vi "Dynamixel Read Pos.vi"(11 "Com port":refnum<visa-resource-name> caption="instrument handle") -> ()   [LabVIEW 2022 SP3]
uses:
  Library/dxl_x64_c.lvlib
  Sub Vis/Dynamixel Commands.ctl
panel:
  in  "Function":T1
  out "value : PRO (knob)\npresent position":i32(knob) scale=150000.0..-150000.0
  in  "protocol_version":i32=2
  out "port_num":i32
  in  "dynamixel_id":u8=1
  in  "baud_rate":i32=57600
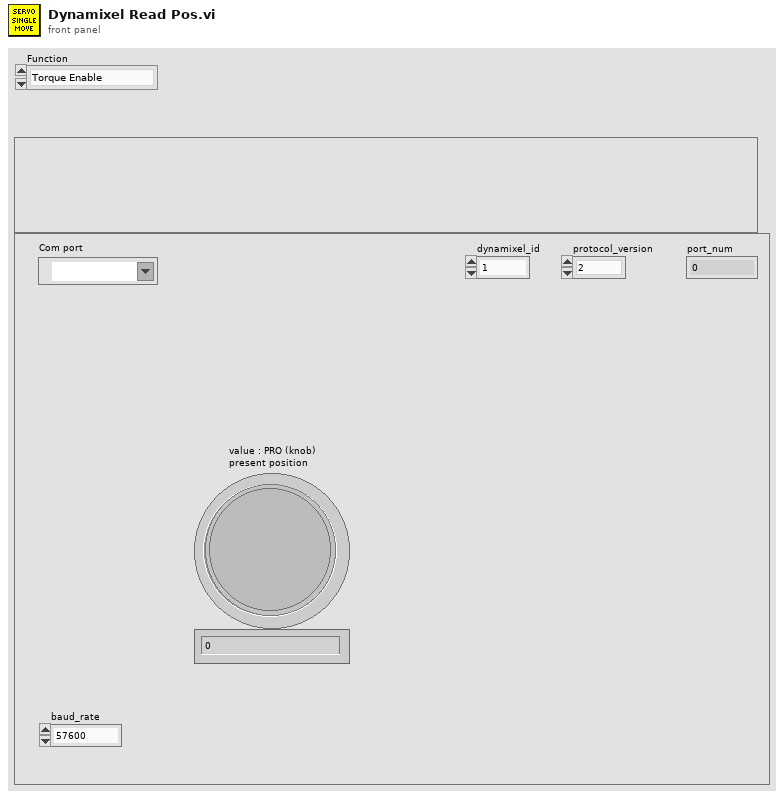
[diagram p1: front panel]
types:
  T1 = typedef "Dynamixel Commands.ctl" = enum16{"Torque Enable", "Present Position", "Threshold", "Max Position Limit", "Acceleration Profile", "Velocity Profile", "Goal Position", "Position Proportional Gain", "Position Integral Gain", "Position Differential Gain ", "Shutdown"}
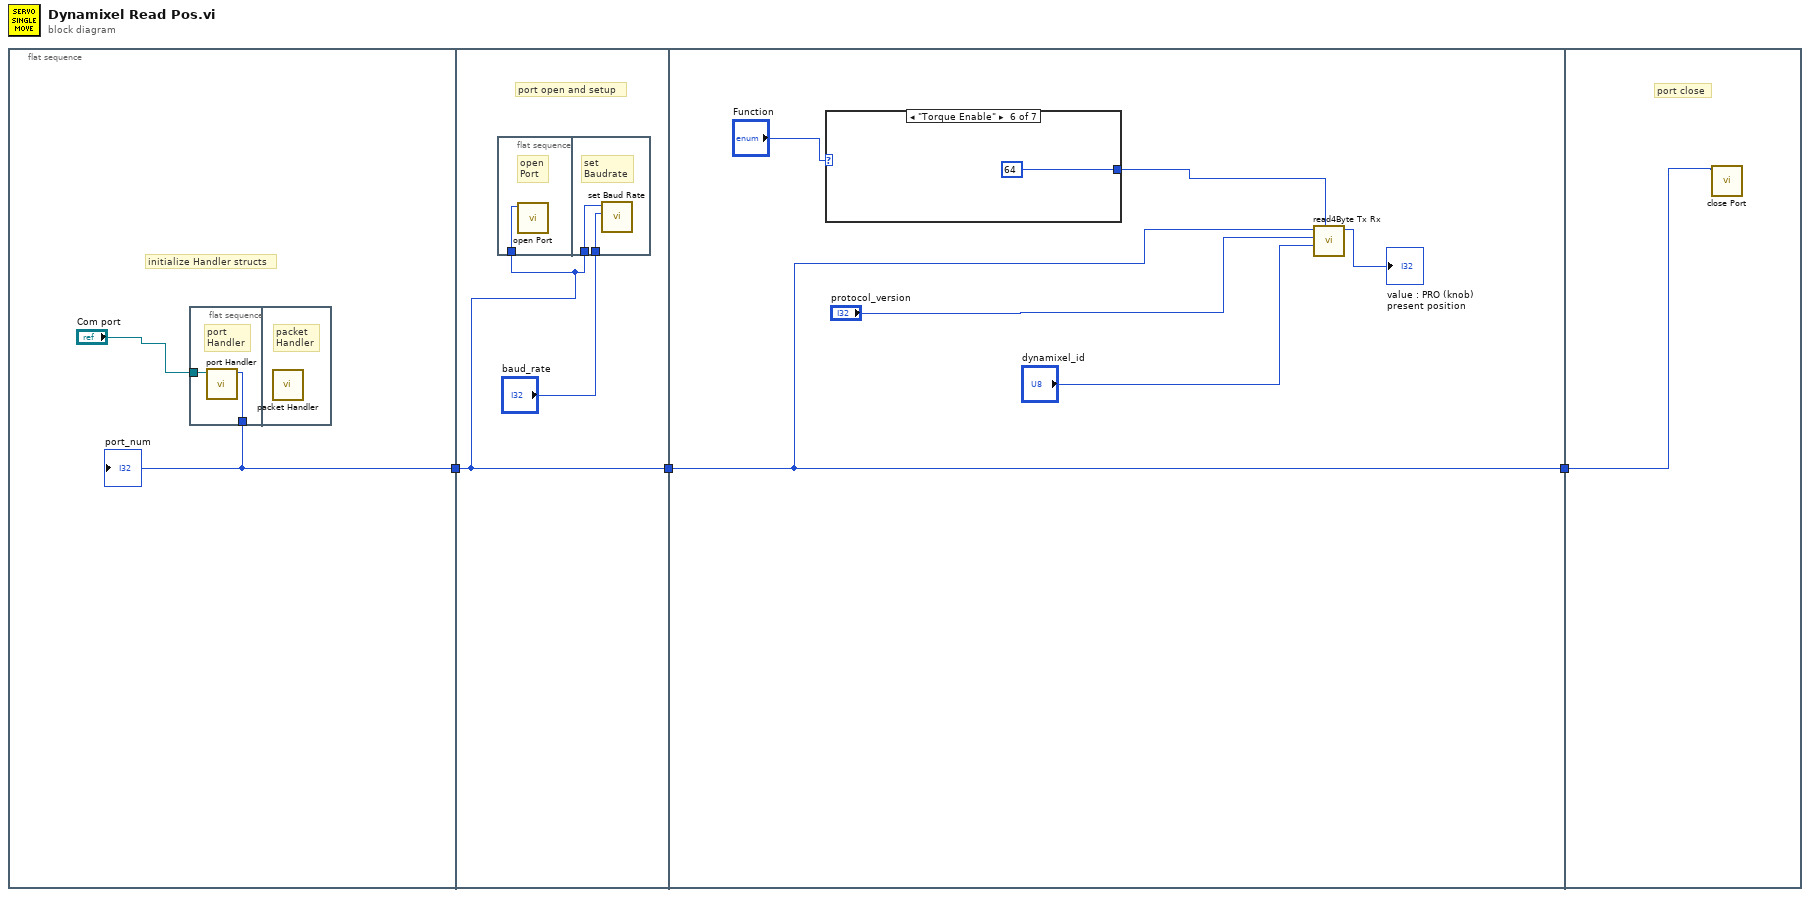
[diagram p0: block diagram]
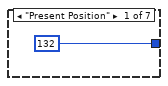
[diagram p2: hidden frame]
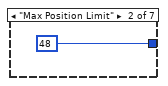
[diagram p3: hidden frame]
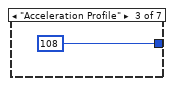
[diagram p4: hidden frame]
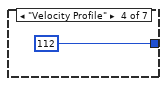
[diagram p5: hidden frame]
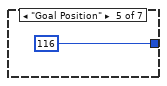
[diagram p6: hidden frame]
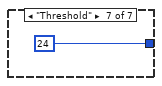
[diagram p7: hidden frame]
diagram:
  n1 = flat-sequence {
    tunnel: [w4] -> w2
    tunnel: [w8] -> w3
    tunnel: w2 -> [w8]
    tunnel: w3 -> [w15]
    tunnel: [w15] -> w1
    tunnel: w1 -> [w26]
    frame #0 {
      # "initialize Handler structs"
      n2 = flat-sequence {
        tunnel: [w7] -> w4
        tunnel: "Com port" -> [w6]
        frame #0 {
          # "port\nHandler"
          n3 = call "port Handler.vi"("port_name"=w6) -> ("function return"=w7:i32)  [unwired: 9 in, 1 out]
        }
        frame #1 {
          # "packet\nHandler"
          n4 = call "packet Handler.vi"() -> ()  [unwired: 11 in, 1 out]
        }
      }
      "port_num" <- w4
    }
    frame #1 {
      # "port open and setup"
      n5 = flat-sequence {
        tunnel: w8 -> [w10]
        tunnel: w8 -> [w12]
        tunnel: "baud_rate" -> [w11]
        frame #0 {
          # "open\nPort"
          n6 = call "open Port.vi"("port_num"=w10) -> ()  [unwired: 9 in, 2 out]
        }
        frame #1 {
          # "set\nBaudrate"
          n7 = call "set Baud Rate.vi"("baudrate"=w11, "port_num"=w12) -> ()  [unwired: 8 in, 2 out]
        }
      }
    }
    frame #2 {
      n8 = case shown="\"Torque Enable\"" "Function" {
        tunnel: [u16 132 ("ADDR_PRO_\nPRESENT_POSITION") u16 48 ("ADDR_PRO_\nPRESENT_POSITION") u16 108 ("ADDR_PRO_\nPRESENT_POSITION") u16 112 ("ADDR_PRO_\nPRESENT_POSITION") u16 116 ("ADDR_PRO_\nPRESENT_POSITION") u16 64 ("ADDR_PRO_\nPRESENT_POSITION") u16 24 ("ADDR_PRO_\nPRESENT_POSITION")] -> w13
        frame "Present Position" {
        }
        frame "Max Position Limit" {
        }
        frame "Acceleration Profile" {
        }
        frame "Velocity Profile" {
        }
        frame "Goal Position" {
        }
        frame "Torque Enable" {
        }
        frame "Threshold" {
        }
      }
      n9 = call "read4Byte Tx Rx.vi"("address"=w13, "id"="dynamixel_id", "protocol_version"="protocol_version", "port_num"=w15) -> ("function return"=→"value : PRO (knob)\npresent position":u32)  [unwired: 6 in, 1 out]
    }
    frame #3 {
      # "port close"
      n10 = call "close Port.vi"("port_num"=w26) -> ()  [unwired: 10 in, 1 out]
    }
  }
